vi "to_U32.vi"(8 "error_in":errorcluster, 10 "variable_start_index":i32, 11 "byte_array":u8[](array[numeric])) -> (0 "error_out":errorcluster, 3 "U32":u32)   [LabVIEW 2020]
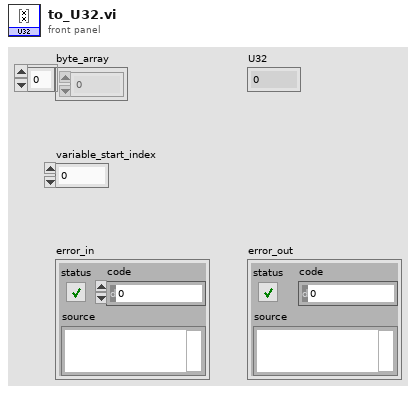
[diagram p1: front panel]
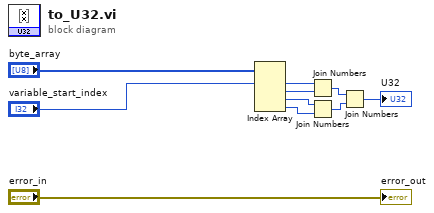
[diagram p0: block diagram]
diagram:
  n1 = Index Array(array="byte_array", index #1="variable_start_index") -> (element #1=w9:u8, element #2=w10:u8, element #3=w6:u8, element #4=w5:u8)  [unwired: 3 in]
  n2 = Join Numbers(hi=w9, lo=w10) -> ((hi.lo)=w4:u16)
  n3 = Join Numbers(hi=w6, lo=w5) -> ((hi.lo)=w3:u16)
  n4 = Join Numbers(hi=w4, lo=w3) -> ((hi.lo)=→"U32":u32)
  "error_out" <- "error_in"
